vi "Make Names.vi"(6 "error in (no error)":errorcluster, 9 "Timetraces in":T1[](array[typedef])) -> (0 "error out":errorcluster, 3 "Names out":string[](array[string]))   [LabVIEW 2009, in "Waveform.lvlib"]
uses:
  Waveform.lvlib
  interface/Timetrace.ctl
  interface/Data Source.ctl
  interface/Interface.lvlib
panel:
  in  "Conflict count":i32
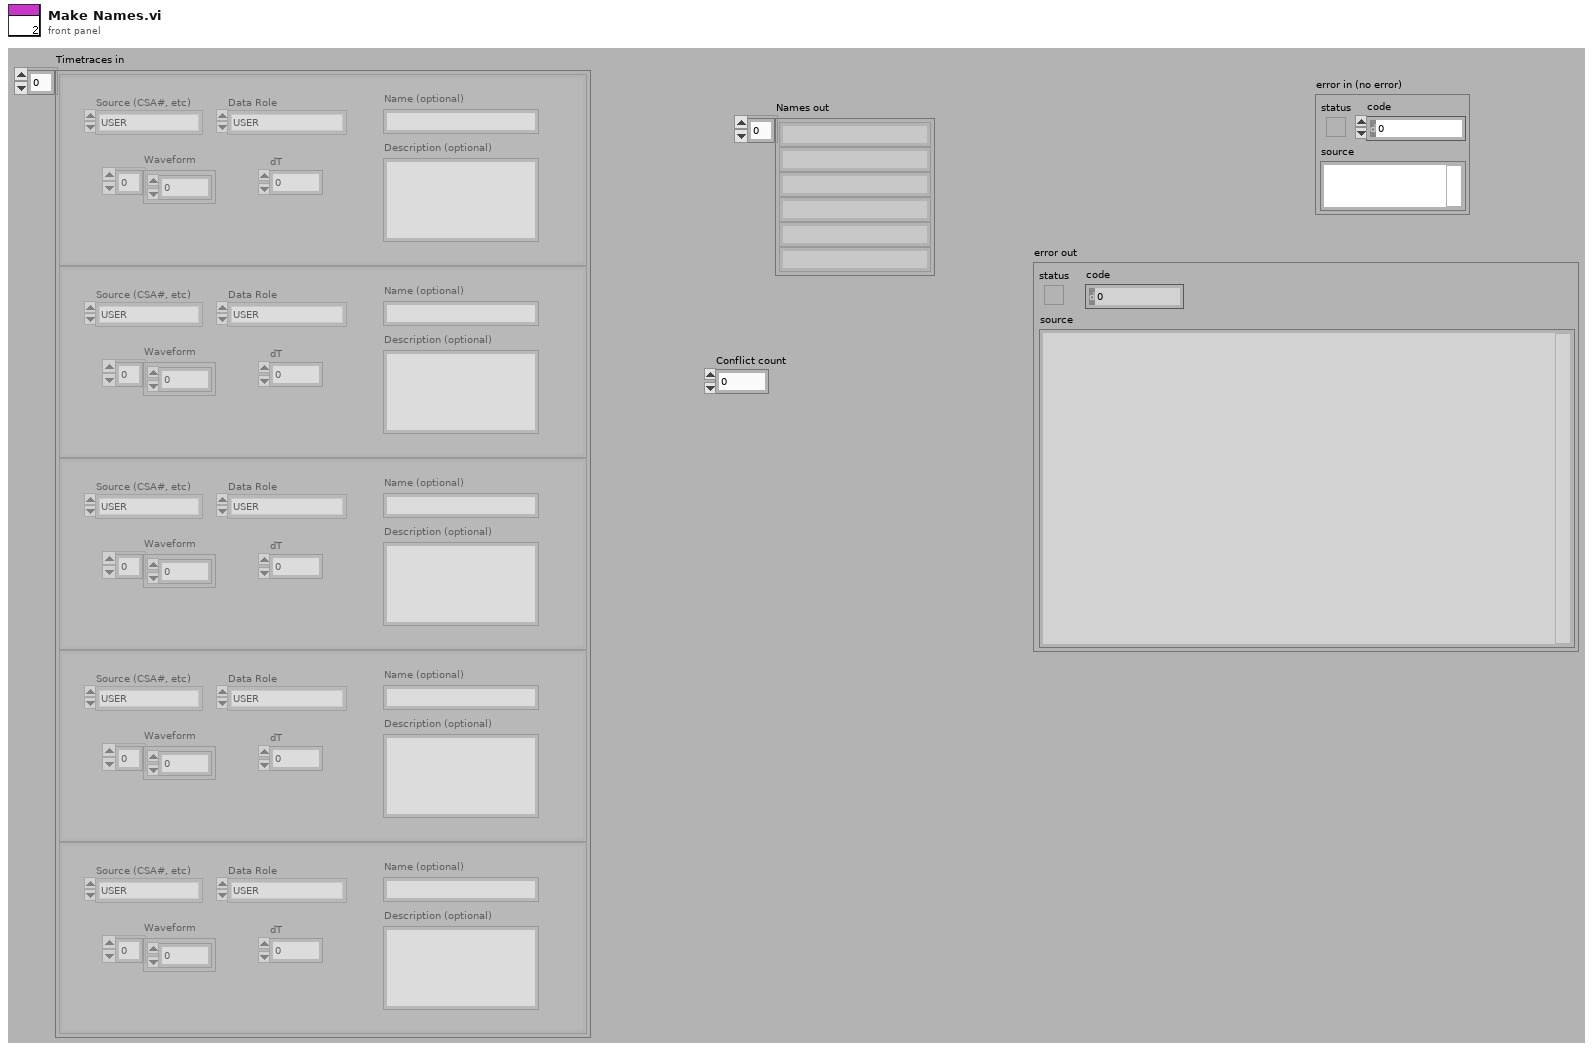
[diagram p1: front panel]
types:
  T1 = typedef "Interface.lvlib/Timetrace.ctl" = cluster{"Source (CSA#, etc)":T2, "Data Role":enum16{"USER", "FIRST DETECTOR", "SECOND DETECTOR", "THIRD DETECTOR", "FINAL DETECTOR"}, "Waveform":sgl[], "dT":sgl, "Name (optional)":string, "Description (optional)":string}
  T2 = typedef "Interface.lvlib/Data Source.ctl" = enum16{"USER", "CSA1", "CSA2", "CSA3", "CSA4", "CSA5", "CSA6", ""}
  T3 = enum16{"USER", "FIRST DETECTOR", "SECOND DETECTOR", "THIRD DETECTOR", "FINAL DETECTOR"}
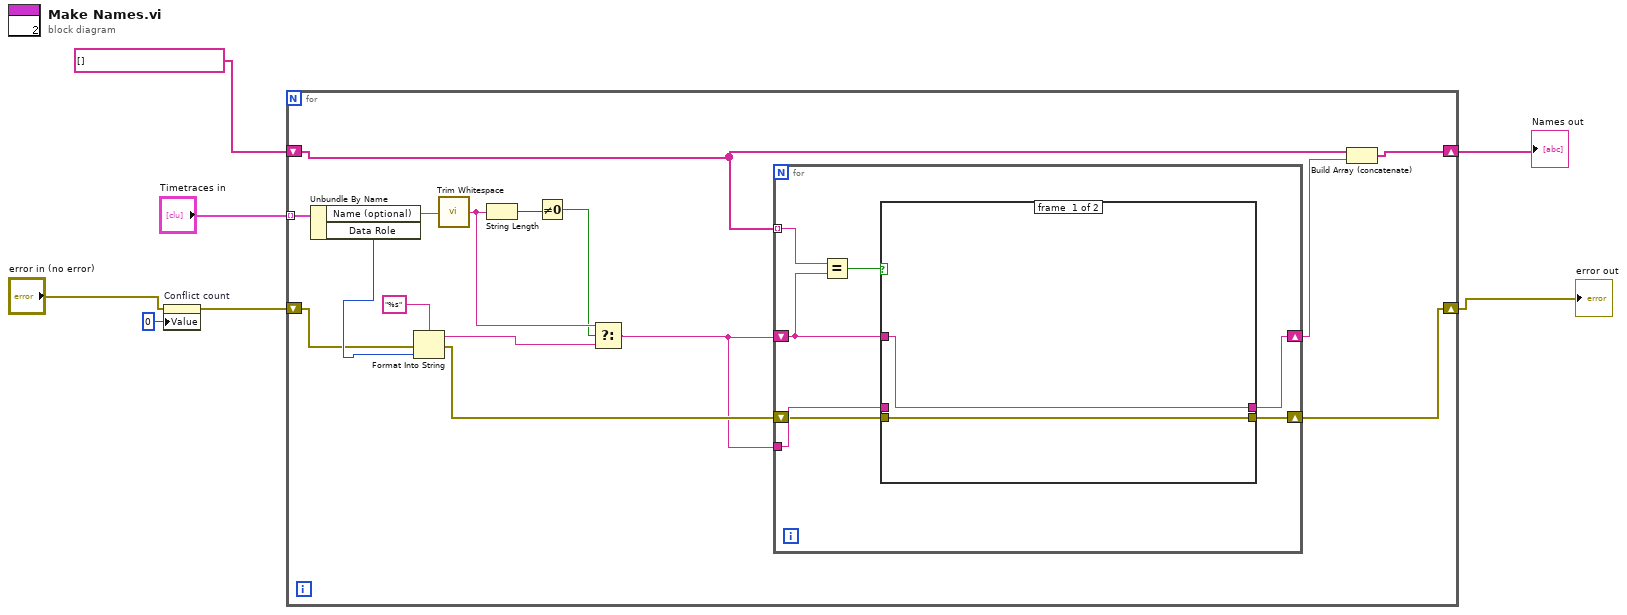
[diagram p0: block diagram]
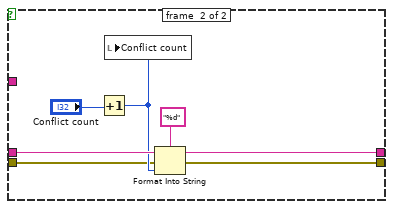
[diagram p2: hidden frame]
diagram:
  n1 = property on="Conflict count" class="DigNum (strict)"(error in="error in (no error)", "Value"=0 ("Conflict count")) -> (error out=w3:errorcluster)  [unwired: 1 in, 1 out]
  n2 = for {
    tunnel: "Timetraces in" -> [w22] mode=indexing
    shift-right: [w16] -> w5
    shift-left: string[] [] -> [w17]
    shift-right: [w13] -> w1
    shift-left: w3 -> [w15]
    n3 = Unbundle By Name(w22) -> ("Name (optional)"=w21:string, "Data Role"=w19:T3)
    n4 = Format Into String(format string="%s", error in=w15, w19) -> (resulting string=w9:string, error out=w14:errorcluster)  [unwired: 1 in]
    n5 = call <vilib>:"Trim Whitespace.vi"("string"=w21) -> ("trimmed string"=w10:string)  [unwired: 1 in]
    n6 = String Length(string=w10) -> (length=w20:i32)
    n7 = Not Equal To 0?(x=w20) -> (x != 0?=w8:bool)
    n8 = Select(t=w10, s=w8, f=w9) -> (s? t:f=w11:string)
    n9 = for {
      tunnel: w17 -> [w29] mode=indexing
      shift-right: [w25] -> w12
      shift-left: w11 -> [w26]
      tunnel: w11 -> [w27]
      shift-right: [w23] -> w13
      shift-left: w14 -> [w24]
      n10 = Equal?(x=w29, y=w26) -> (x = y?=w28:bool)
      n11 = case shown="True" w28 {
        tunnel: w27 -> [_ w37]
        tunnel: w26 -> [w31 _]
        tunnel: [w31 w34] -> w25
        tunnel: w24 -> [w30 w33]
        tunnel: [w30 w32] -> w23
        frame #0 {
        }
        frame #1 {
          n12 = Increment(x="Conflict count") -> (x+1=w35:i32)
          n13 = local write "Conflict count"(w35) -> ()
          n14 = Format Into String(format string="%d", initial string=w37, error in=w33, w35) -> (resulting string=w34:string, error out=w32:errorcluster)
        }
      }
    }
    n15 = Build Array (concatenate)(w17, w12) -> (w16:string[])
  }
  "Names out" <- w5
  "error out" <- w1
